vi "Setup.vi"(8 "error in (no error)":errorcluster) -> (0 "error out":errorcluster)   [LabVIEW 2011]
uses:
  090 - ERRORS/Ctrls/EnumErrors.ctl
  050 - CONFIG/00 - ApplicationConfig/Ctrls/EnumFgvConfigCommand.ctl
  030 - EVENTS/EnumFgvEventCommand.ctl
  100_PROCESS/SubVis/EnumFgvReferenceProcess.ctl
  100_PROCESS/EnumProcess.ctl
  030 - EVENTS/03 - ToMessageHandlerProcess/enumMessageCriticity.ctl
  090 - ERRORS/Ctrls/enumLogAndView.ctl
panel:
  # "SETUP"
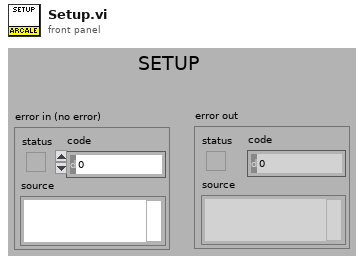
[diagram p1: front panel]
types:
  T1 = typedef "EnumErrors.ctl" = enum16{"VI non trouvé !", "Clé non trouvée", "Timeout", "Le VI tourne déjà", "Erreur de séparateur décimal", "Référence non trouvée"}
  T2 = typedef "EnumFgvConfigCommand.ctl" = enum16{"Load", "Get", "Set", "Save To Disk"}
  T3 = typedef "EnumFgvReferenceProcess.ctl" = enum16{"Init", "Get", "Add Reference", "Close References"}
  T4 = typedef "EnumProcess.ctl" = enum16{"Message handler", "Template"}
  T5 = typedef "enumMessageCriticity.ctl" = enum16{"No error", "Info", "Warning", "Error", "Fatal error"}
  T6 = typedef "enumLogAndView.ctl" = enum16{"Log only", "Log and view"}
  T7 = typedef "BenchConfig.ctl" = cluster{"Cfg":string}
  T8 = typedef "EnumFgvEventCommand.ctl" = enum16{"Setup", "Cleanup", "Get"}
  T9 = typedef "paramsExternalProcesses.ctl" = cluster{"File Path Control":path, "Timeout":dbl, "viInitString":string, "State":enum32{"Invalid", "Standard", "Closed", "Hidden", "Minimized", "Maximized"}}
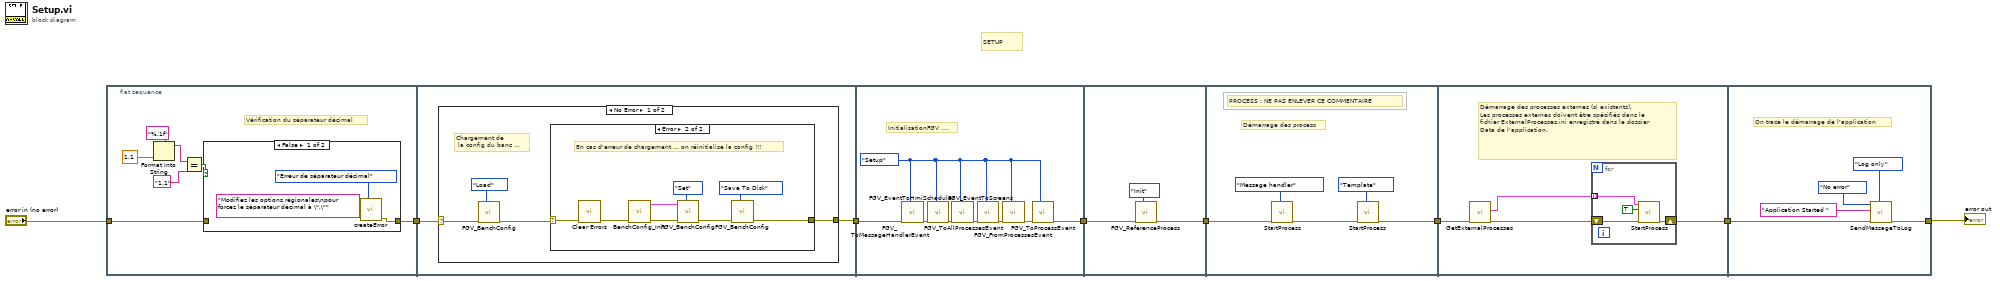
[diagram p0: block diagram]
diagram:
  # "SETUP"
  n1 = flat-sequence {
    tunnel: "error in (no error)" -> [w10]
    tunnel: [w9] -> w5
    tunnel: [w21] -> w6
    tunnel: w5 -> [w20]
    tunnel: w6 -> [w42]
    tunnel: [w37] -> w2
    tunnel: w2 -> [w46]
    tunnel: [w45] -> w1
    tunnel: w1 -> [w51]
    tunnel: [w47] -> w3
    tunnel: [w55] -> w4
    tunnel: w3 -> [w52]
    tunnel: [w64] -> w7
    tunnel: w4 -> [w60]
    frame #0 {
      # "Vérification du séparateur décimal"
      n2 = Format Into String(format string="%.1f", 1.1) -> (resulting string=w13:string)  [unwired: 2 in, 1 out]
      n3 = Equal?(x=w13, y="1.1") -> (x = y?=w11:bool)
      n4 = case shown="False" w11 {
        tunnel: w10 -> [_ w19]
        tunnel: [w18 w19] -> w9
        frame False {
          n5 = call "createError.vi"("ErrorCode"=EnumErrors."Erreur de séparateur décimal", "message"="Modifiez les options régionales\npour forcez le séparateur décimal à \".\"") -> ("error out"=w18:errorcluster)  [unwired: 9 in]
        }
        frame True {
        }
      }
    }
    frame #1 {
      n6 = case shown="No Error" w20 {
        selector: w20 -> [w25 w35]
        tunnel: [w22 w35] -> w21
        frame No Error {
          # "Chargement de\n la config du banc ..."
          n7 = call "FGV_BenchConfig.vi"("Command"=EnumFgvConfigCommand."Load", "error in (no error)"=w25) -> ("error out"=w23:errorcluster)  [unwired: 8 in, 1 out]
          n8 = case shown="Error" w23 {
            selector: w23 -> [w26 w29]
            tunnel: [w26 w28] -> w22
            frame No Error {
            }
            frame Error {
              # "En cas d'erreur de chargement ... on réinitialise la config !!!"
              n9 = call <vilib>:"Clear Errors.vi"("error in (no error)"=w29) -> ("error out"=w27:errorcluster)  [unwired: 6 in]
              n10 = call "BenchConfig_Init.vi"("error in (no error)"=w27) -> ("error out"=w32:errorcluster, "BenchConfig"=w33:T7)  [unwired: 9 in]
              n11 = call "FGV_BenchConfig.vi"("Command"=EnumFgvConfigCommand."Set", "error in (no error)"=w32, "BenchConfigIn"=w33) -> ("error out"=w30:errorcluster)  [unwired: 7 in, 1 out]
              n12 = call "FGV_BenchConfig.vi"("Command"=EnumFgvConfigCommand."Save To Disk", "error in (no error)"=w30) -> ("error out"=w28:errorcluster)  [unwired: 8 in, 1 out]
            }
          }
        }
        frame Error {
        }
      }
    }
    frame #2 {
      w36 = EnumFgvEventCommand."Setup" ("Command")
      # "InitialisationFGV ...."
      n13 = call "FGV_ToMessageHandlerEvent.vi"("Command"=w36, "error in (no error)"=w42) -> ("error out"=w41:errorcluster)  [unwired: 8 in, 1 out]
      n14 = call "FGV_EventToHmiScheduler.vi"("Command"=w36, "error in (no error)"=w41) -> ("error out"=w43:errorcluster)  [unwired: 8 in, 1 out]
      n15 = call "FGV_EventToScreens.vi"("Command"=w36, "error in (no error)"=w43) -> ("error out"=w40:errorcluster)  [unwired: 8 in, 1 out]
      n16 = call "FGV_ToAllProcessesEvent.vi"("Command"=w36, "error in (no error)"=w40) -> ("error out"=w39:errorcluster)  [unwired: 8 in, 1 out]
      n17 = call "FGV_FromProcessesEvent.vi"("Command"=w36, "error in (no error)"=w39) -> ("error out"=w38:errorcluster)  [unwired: 8 in, 1 out]
      n18 = call "FGV_ToProcessEvent.vi"("Command"=w36, "error in (no error)"=w38) -> ("error out"=w37:errorcluster)  [unwired: 8 in, 1 out]
    }
    frame #3 {
      n19 = call "FGV_ReferenceProcess.vi"("Commande"=EnumFgvReferenceProcess."Init", "error in (no error)"=w46) -> ("error out"=w45:errorcluster)  [unwired: 8 in, 1 out]
    }
    frame #4 {
      # "PROCESS : NE PAS ENLEVER CE COMMENTAIRE"
      # "Démarrage des process"
      n20 = call "StartProcess.vi"("Process"=EnumProcess."Message handler", "error in (no error)"=w51) -> ("error out"=w49:errorcluster)  [unwired: 9 in]
      n21 = call "StartProcess.vi"("Process"=EnumProcess."Template", "error in (no error)"=w49) -> ("error out"=w47:errorcluster)  [unwired: 9 in]
    }
    frame #5 {
      # "Démarrage des processes externes (si existants).\nLes processes externes doivent être spécifiés dans le fichier ExternalProcesses.ini enregistré dans le dossier Data de l'application."
      n22 = call "GetExternalProcesses.vi"("Error In"=w52) -> ("Error Out"=w54:errorcluster, "ExternalProcesses"=w53:T9[])  [unwired: 9 in]
      n23 = for {
        shift-right: [w57] -> w55
        shift-left: w54 -> [w59]
        tunnel: w53 -> [w56] mode=indexing
        n24 = call "StartProcess.vi"("error in (no error)"=w59, "externalProcess?"=TRUE, "viToLaunchInfos"=w56) -> ("error out"=w57:errorcluster)  [unwired: 8 in]
      }
    }
    frame #6 {
      # "On trace le démarrage de l'application"
      n25 = call "SendMessageToLog.vi"("Log and view ?"=enumLogAndView."Log only", "error in (no error)"=w60, "Message"="Application Started ", "Criticity"=enumMessageCriticity."No error") -> ("error out"=w64:errorcluster)  [unwired: 7 in]
    }
  }
  "error out" <- w7
